vi "InteractiveStepperControlDLL.vi"() -> ()   [LabVIEW 2015]
doc: "Commands\n 0 - set units (0-inHg, 1-mmHg, 2-torr, 3-mbar)\n 1 - set vacuum zero\n 2 - reserved\n 3 - reserved\n 4 - reserved\n 5 - set vacuum calibration\n 6 - reserved\n 7 - start bootloader\n 8 - get firmware version\n 9 - get vacuum reading\n 10 - start/stop vacuum control (0-stop, 1-start)\n 11 - set vacuum setpoint\n 12 - set calibration zero offset (prevent negative zero value from DWIN)\n 13 - set pump speed 0-100 \n 14 - set vacuum valve PWM 0-1000\n 15 - set bleed valve PWM 0-1000"
uses:
  C:/_User/GitHub Projects/PulseGen/StepperDLL/StepperDLL/bin/Debug/StepperDLL.dll
  StepperDLL/StepperDLL/bin/Debug/StepperDLL.dll
panel:
  in  "Move":bool
  in  "Hz":sgl=1.0 min=1 max=2000 step=1
  in  "Steps":sgl min=0 max=100000 step=1
  in  "Direction":bool
  in  "Enable":bool
  in  "stop":bool
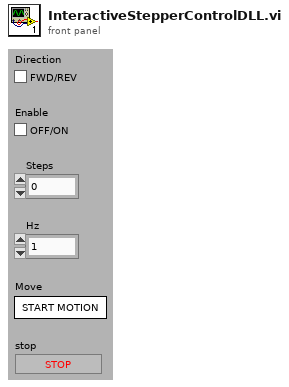
[diagram p1: front panel]
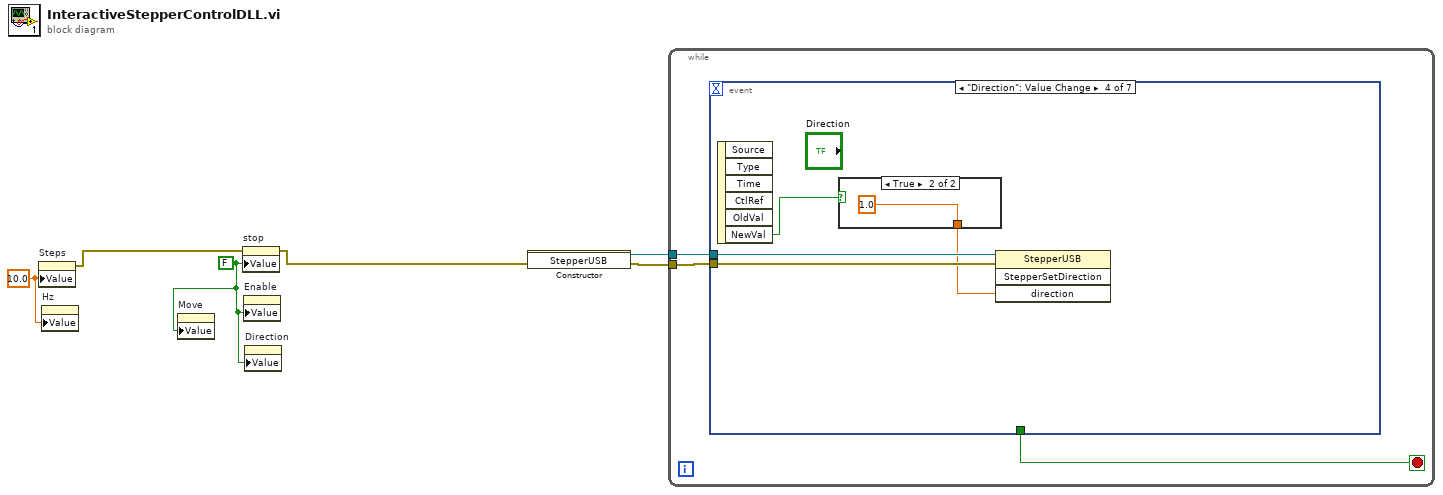
[diagram p0: block diagram]
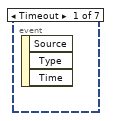
[diagram p2: hidden frame]
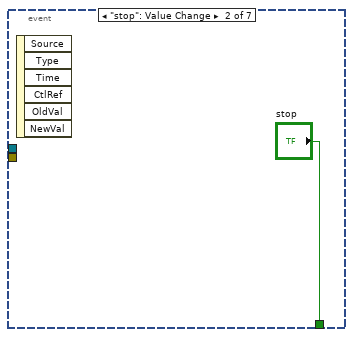
[diagram p3: hidden frame]
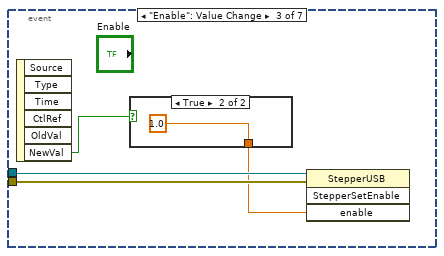
[diagram p4: hidden frame]
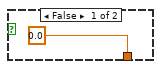
[diagram p5: hidden frame]
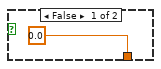
[diagram p6: hidden frame]
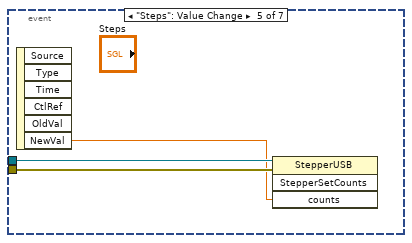
[diagram p7: hidden frame]
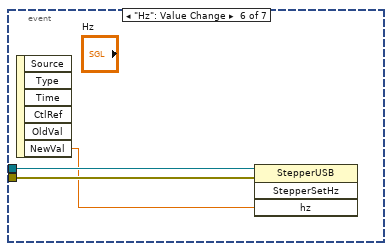
[diagram p8: hidden frame]
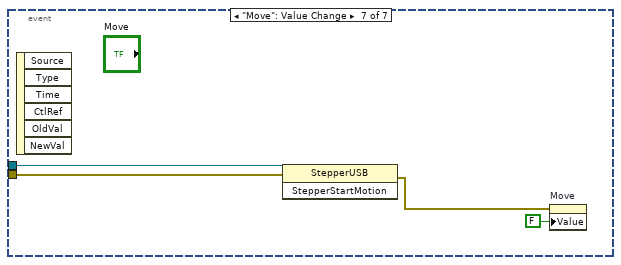
[diagram p9: hidden frame]
diagram:
  w6 = sgl 10.0 ("Steps")
  w5 = FALSE ("stop")
  n1 = property on="Steps" class="DigNum (strict)"("Value"=w6) -> (error out=w2:errorcluster)  [unwired: 2 in, 1 out]
  n2 = property on="Hz" class="DigNum (strict)"("Value"=w6) -> ()  [unwired: 2 in, 2 out]
  n3 = property on="Move" class="Bool (strict)"("Value"=w5) -> ()  [unwired: 2 in, 2 out]
  n4 = property on="stop" class="Bool (strict)"(error in=w2, "Value"=w5) -> (error out=w1:errorcluster)  [unwired: 1 in, 1 out]
  n5 = property on="Enable" class="Bool (strict)"("Value"=w5) -> ()  [unwired: 2 in, 2 out]
  n6 = property on="Direction" class="Bool (strict)"("Value"=w5) -> ()  [unwired: 2 in, 2 out]
  n7 = constructor class="StepperUSB"(error in=w1) -> (reference out=w4:refnum<k24>, error out=w3:errorcluster)  [unwired: 2 in, 1 out]
  n8 = while {
    tunnel: w4 -> [w8]
    tunnel: w3 -> [w7]
    stop <- w9 stop-if-true
    n9 = event shown="[3] \"Direction\": Value Change" {
      selector: _ -> [_ _ _ _ _ _ _]
      dyn-events: _ -> [_ _ _ _ _ _ _]
      timeout: _ -> [_ _ _ _ _ _ _]
      tunnel: [_ "stop" _ _ _ _ _] -> w9
      tunnel: w8 -> [_ _ w13 w19 w25 w28 w31]
      tunnel: w7 -> [_ _ w12 w18 w24 w27 w30]
      event Timeout {
        n10 = event-data() -> ()  [unwired: 1 in, 3 out]
      }
      event "stop": Value Change {
        n11 = event-data() -> ()  [unwired: 1 in, 6 out]
      }
      event "Enable": Value Change {
        n12 = event-data() -> ("NewVal"=w14:bool)  [unwired: 1 in, 5 out]
        n13 = case shown="True" w14 {
          tunnel: [sgl 0.0 sgl 1.0] -> w11
          frame False {
          }
          frame True {
          }
        }
        n14 = invoke class="StepperUSB" method="StepperSetEnable"(reference=w13, error in=w12, "enable"=w11) -> ()  [unwired: 1 in, 4 out]
      }
      event "Direction": Value Change {
        n15 = event-data() -> ("NewVal"=w20:bool)  [unwired: 1 in, 5 out]
        n16 = case shown="True" w20 {
          tunnel: [sgl 0.0 sgl 1.0] -> w17
          frame False {
          }
          frame True {
          }
        }
        n17 = invoke class="StepperUSB" method="StepperSetDirection"(reference=w19, error in=w18, "direction"=w17) -> ()  [unwired: 1 in, 4 out]
      }
      event "Steps": Value Change {
        n18 = event-data() -> ("NewVal"=w23:sgl)  [unwired: 1 in, 5 out]
        n19 = invoke class="StepperUSB" method="StepperSetCounts"(reference=w25, error in=w24, "counts"=w23) -> ()  [unwired: 1 in, 4 out]
      }
      event "Hz": Value Change {
        n20 = event-data() -> ("NewVal"=w26:sgl)  [unwired: 1 in, 5 out]
        n21 = invoke class="StepperUSB" method="StepperSetHz"(reference=w28, error in=w27, "hz"=w26) -> ()  [unwired: 1 in, 4 out]
      }
      event "Move": Value Change {
        n22 = event-data() -> ()  [unwired: 1 in, 6 out]
        n23 = invoke class="StepperUSB" method="StepperStartMotion"(reference=w31, error in=w30) -> (error out=w29:errorcluster)  [unwired: 1 in, 2 out]
        n24 = property on="Move" class="Bool (strict)"(error in=w29, "Value"=FALSE ("Move")) -> ()  [unwired: 1 in, 2 out]
      }
    }
  }
